vi "Filter.vi"(8 "error in (no error)":errorcluster, 11 "Software Lock-in in":refnum<class "Software Lock-in.lvclass">) -> (0 "error out":errorcluster, 3 "Software Lock-in out":refnum<class "Software Lock-in.lvclass">)   [LabVIEW 2015, in "Software Lock-in.lvclass"]
uses:
  Software Lock-in.lvclass
  Software Lock-in.lvclass/Software Lock-in.ctl
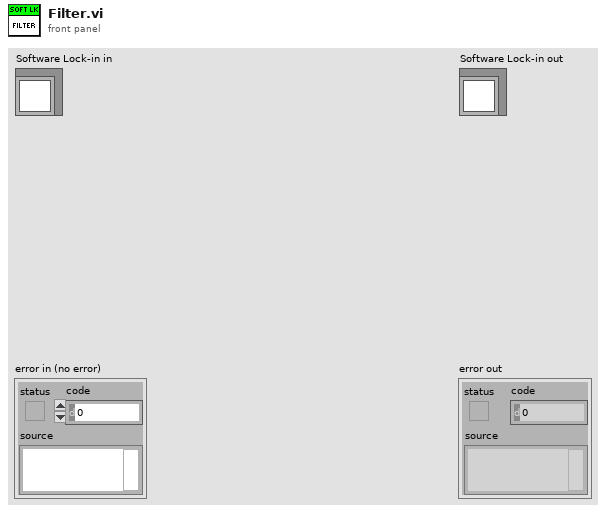
[diagram p1: front panel]
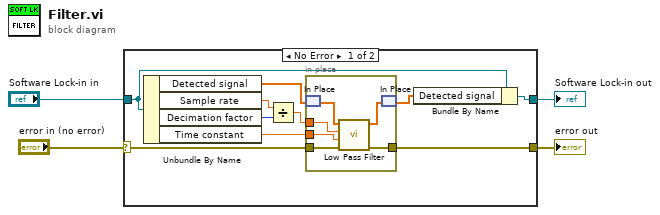
[diagram p0: block diagram]
diagram:
  n1 = case shown="No Error" "error in (no error)" {
    selector: "error in (no error)" -> [w7 w22]
    tunnel: [w6 w22] -> w3
    tunnel: [w9 w21] -> w1
    tunnel: "Software Lock-in in" -> [w14 w21]
    frame No Error {
      n2 = Unbundle By Name(w14) -> ("Detected signal"=w13:cdb[], "Sample rate"=w12:dbl, "Decimation factor"=w11:i32, "Time constant"=w5:dbl)
      n3 = Divide(x=w12, y=w11) -> (x/y=w10:dbl)
      n4 = in-place {
        in-place-border: w10 -> [w15]
        in-place-border: w7 -> [w20]
        in-place-border: [w19] -> w6
        in-place-border: w5 -> [w16]
        n5 = in-place-match #1(w13) -> (w18:cdb[])
        n6 = call "Low Pass Filter.vi"("Error In"=w20, "Time constant"=w16, "Saple rate"=w15, "Data"=w18) -> ("Error Out"=w19:errorcluster, "Data out"=w17:cdb[])  [unwired: 6 in]
        n7 = in-place-match #1(w17) -> (w8:cdb[])
      }
      n8 = Bundle By Name(cluster=w14, "Detected signal"=w8) -> (w9:refnum<class "Software Lock-in.lvclass">)
    }
    frame Error {
    }
  }
  "error out" <- w3
  "Software Lock-in out" <- w1
